vi "Main.vi"() -> ()   [LabVIEW 2020]
doc: "This template is for the Queued Message Handler design pattern.\n\nThe Event Handling Loop generates messages based on user interface actions.\n\nThe Message Handling Loop processes messages generated by the Event Handling Loop, or by other messages. The messages are string values, so new messages can be added easily to the Message Cases case structure in the Message Handling Loop. Each message cluster can also provide an optional value for Message Data, which is a variant that can be converted to whatever message-specific data is required."
uses:
  controls/UI Data.ctl
  controls/Timer Status.ctl
  <vilib>/Skyline/Message/HTTP Wrapper/NI Skyline Message HTTP.lvclass
  C:/Program Files (x86)/National Instruments/LabVIEW 2020/vi.lib/Skyline/Message/NI Skyline Message.lvclass
  <vilib>/Skyline/Configuration/Configuration HTTP_class/Open Configuration HTTP.vi
  <vilib>/Utility/error.llb/Error Cluster From Error Code.vi
  support/Message Queue/Enqueue Message (Single).vi
  <vilib>/ErrorRing/Error Ring.xnode
  support/Message Queue/Message Queue.lvlib
  support/User Event - Stop/User Event - Stop.lvlib
  <vilib>/Skyline/Configuration/Configuration HTTP_class/NI Skyline Configuration HTTP.lvclass
panel:
  in  "Reset Button":bool
  in  "Pause Button":bool
  in  "Start Button":bool
  out "Running":bool
  out "Timer":dbl format="%.2f"
  in  "Exit":bool
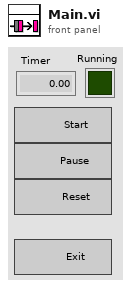
[diagram p1: front panel]
types:
  T1 = typedef "UI Data.ctl" = cluster{"Start":dbl, "Accumulated":dbl, "Running":bool}
  T2 = typedef "Message Queue.lvlib/All Message Queues.ctl" = cluster{"UI":refnum<queue>}
  T3 = typedef "Timer Status.ctl" = cluster{"Elapsed":dbl, "Running":bool}
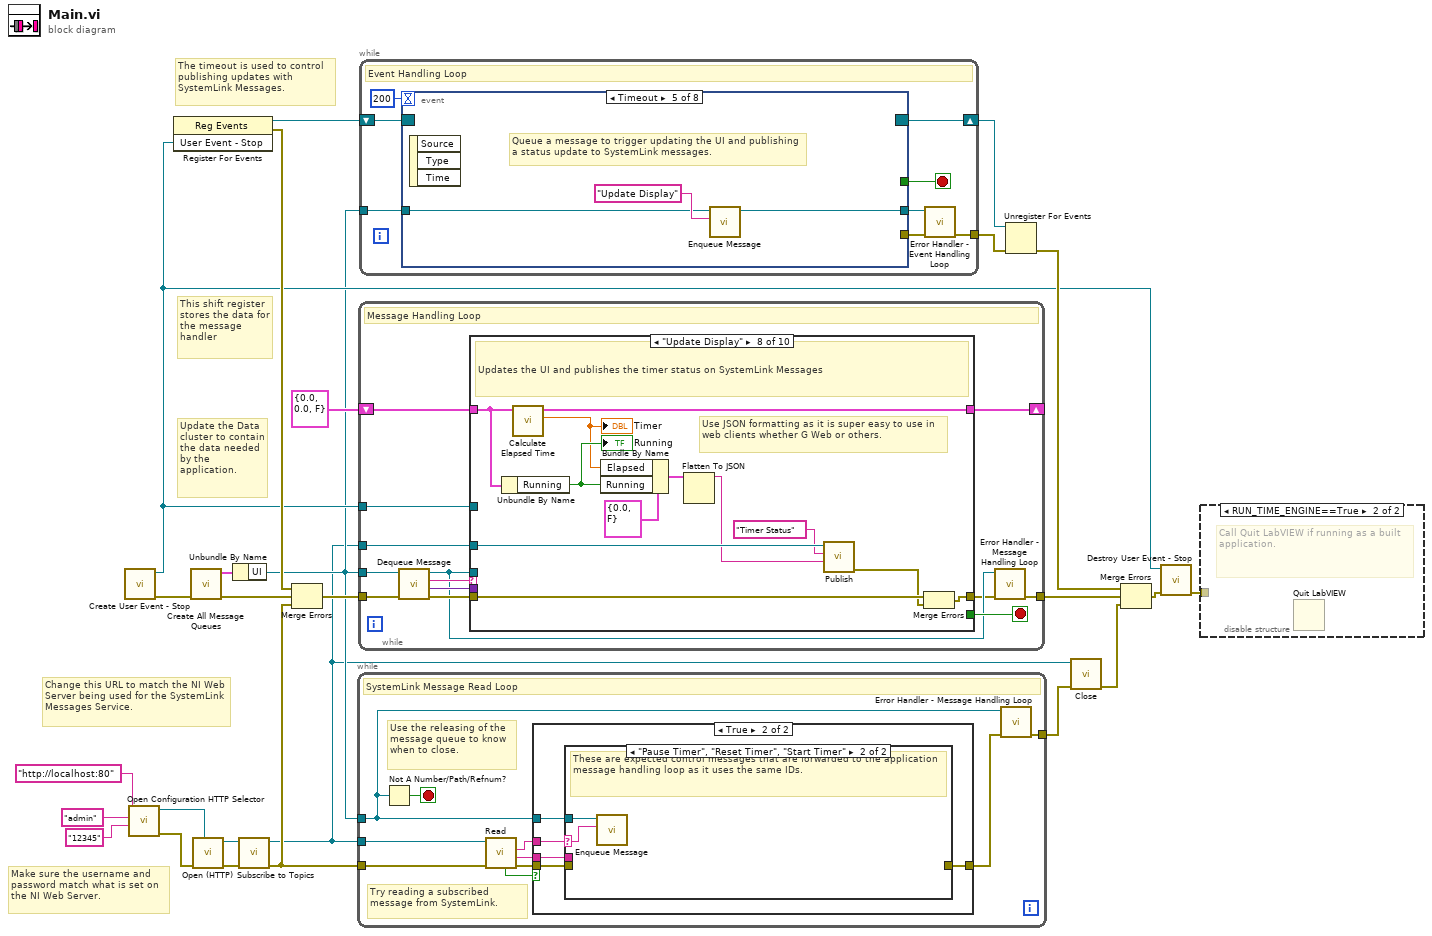
[diagram p0: block diagram]
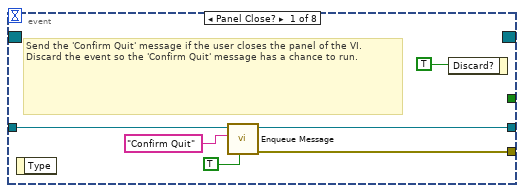
[diagram p3: hidden frame]
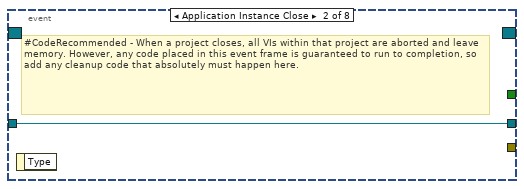
[diagram p4: hidden frame]
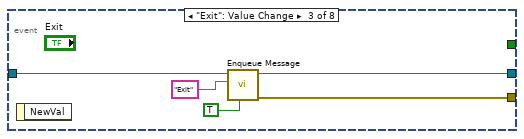
[diagram p5: hidden frame]
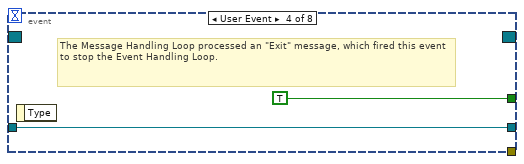
[diagram p6: hidden frame]
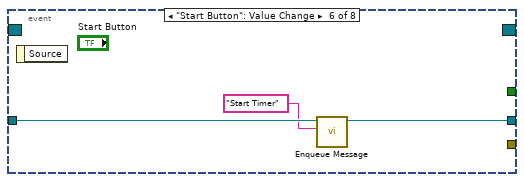
[diagram p7: hidden frame]
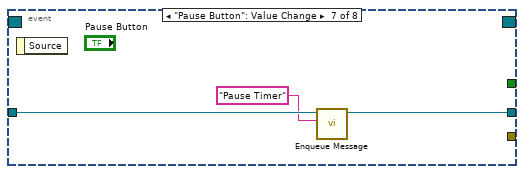
[diagram p8: hidden frame]
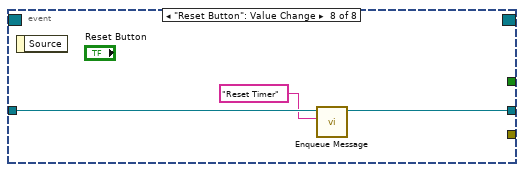
[diagram p9: hidden frame]
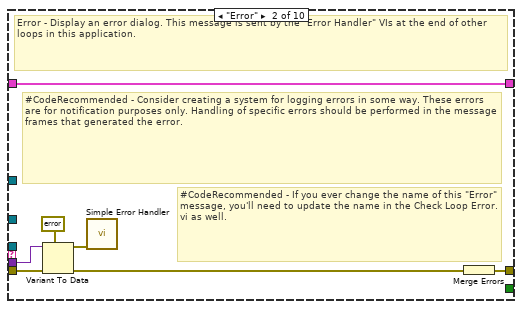
[diagram p11: hidden frame]
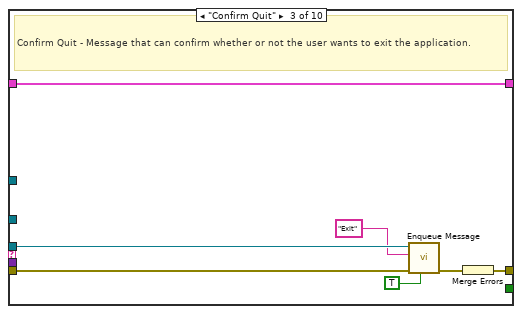
[diagram p12: hidden frame]
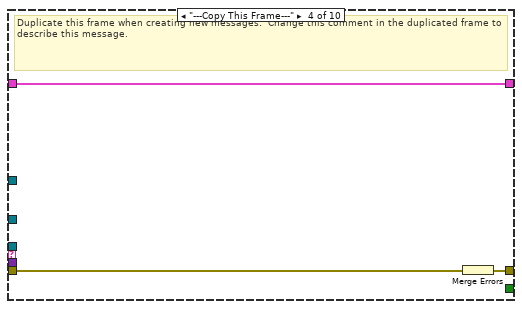
[diagram p13: hidden frame]
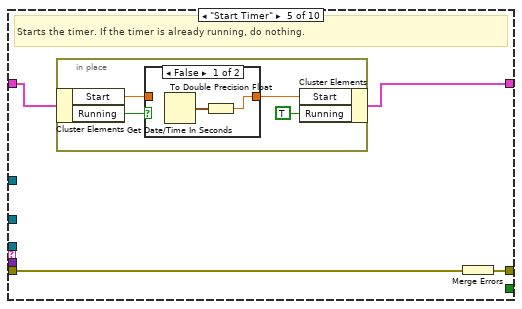
[diagram p14: hidden frame]
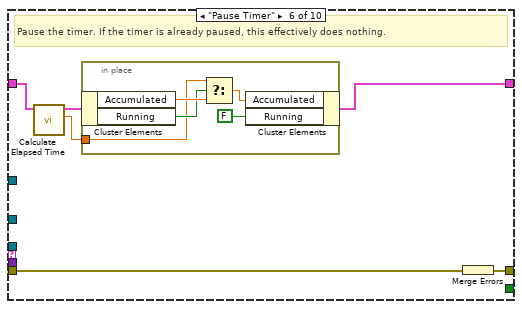
[diagram p16: hidden frame]
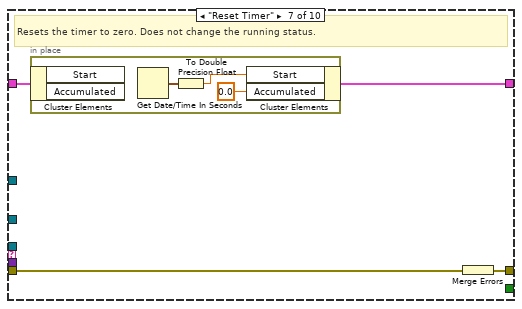
[diagram p17: hidden frame]
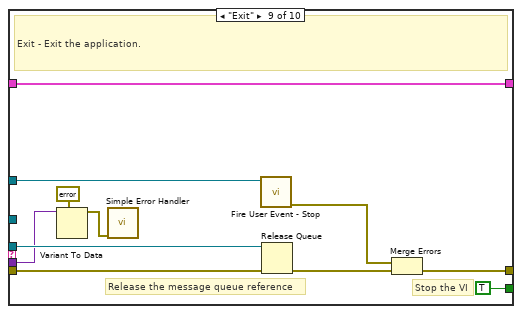
[diagram p18: hidden frame]
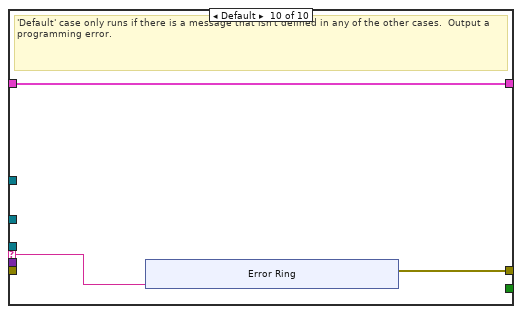
[diagram p19: hidden frame]
diagram:
  # "The timeout is used to control publishing updates with SystemLink Messages."
  # "Update the Data cluster to contain the data needed by the application."
  # "Make sure the username and password match what is set on the NI Web Server."
  # "Change this URL to match the NI Web Server being used for the SystemLink Messages Service."
  # "This shift register stores the data for the message handler"
  n1 = call "Create User Event - Stop.vi"() -> ("error out"=w21:errorcluster, "User Event - Stop"=w13:refnum<user-event>)  [unwired: 10 in]
  n2 = call-poly <vilib>:"Open Configuration HTTP Selector.vi"("password"="12345", "username"="admin", "server url"="http://localhost:80") -> ("error out"=w11:errorcluster, "configuration"=w10:refnum<class "NI Skyline Configuration HTTP.lvclass">)  [unwired: 7 in]
  n3 = register-events(w13) -> (reference out=w14:refnum<event-registration>, error out=w26:errorcluster)  [unwired: 2 in]
  n4 = call "Create All Message Queues.vi"("error in (no error)"=w21) -> ("error out"=w24:errorcluster, "Message Queues out"=w23:T2)  [unwired: 9 in]
  n5 = call <vilib>:"Open (HTTP).vi"("configuration"=w10, "error in (no error)"=w11) -> ("error out"=w6:errorcluster, "message session"=w5:refnum<class "NI Skyline Message HTTP.lvclass">)  [unwired: 8 in]
  n6 = Unbundle By Name(w23) -> ("UI"=w2:refnum<queue>)
  n7 = call "Subscribe to Topics.vi"("error in (no error)"=w6, "message session in"=w5) -> ("error out"=w25:errorcluster, "message session out"=w1:refnum<class "NI Skyline Message HTTP.lvclass">)  [unwired: 8 in]
  n8 = Merge Errors(w26, w24, w25) -> (w12:errorcluster)
  n9 = while {
    tunnel: w2 -> [w28]
    tunnel: w1 -> [w36]
    tunnel: w25 -> [w35]
    tunnel: [w29] -> w4
    stop <- w27 stop-if-true
    # "Try reading a subscribed message from SystemLink."
    # "Use the releasing of the message queue to know when to close."
    # "SystemLink Message Read Loop"
    n10 = Not A Number/Path/Refnum?(number/path/refnum=w28) -> (NaN/Path/Refnum?=w27:bool)
    n11 = call-dynamic "Read.vi"("error in (no error)"=w35, "sync message session in"=w36) -> ("error out"=w31:errorcluster, "message"=w32:string, "topic"=w33:string, "dequeue status"=w34:bool)  [unwired: 5 in, 1 out]
    n12 = case shown="True" w34 {
      tunnel: w33 -> [_ w42]
      tunnel: w32 -> [_ w41]
      tunnel: w28 -> [_ w40]
      tunnel: w31 -> [w37 w39]
      tunnel: [w37 w38] -> w30
      frame False {
        # "No message was received on a topic that's subscribed to, just iterate or possible handle the error that may have been returned from Read.vi"
      }
      frame True {
        n13 = case shown="\"Pause Timer\", \"Reset Timer\", \"Start Timer\"" w42 {
          selector: w42 -> [w43 w52]
          tunnel: w41 -> [_ _]
          tunnel: w40 -> [_ w53]
          tunnel: w39 -> [_ _]
          tunnel: [w44 _] -> w38
          frame Default {
            # "An unrecognized message topic was received. Since we subscribe to specific messages generate an error for the developer to fix."
            n14 = xnode "Error Ring"("parameter 0"=w43) -> ("error out"=w44:errorcluster)
          }
          frame "Pause Timer", "Reset Timer", "Start Timer" {
            # "These are expected control messages that are forwarded to the application message handling loop as it uses the same IDs."
            n15 = call-poly "Enqueue Message.vi"("Message"=w52, "Message Queue"=w53) -> ()  [unwired: 8 in, 2 out]
          }
        }
      }
    }
    n16 = call "Error Handler - Message Handling Loop.vi"("error in (no error)"=w30, "Message Queue"=w28) -> ("dup error in"=w29:errorcluster)  [unwired: 8 in, 1 out]
  }
  n17 = while {
    tunnel: w2 -> [w58]
    shift-right: [w65] -> _
    shift-left: T1 {"Start"=0.0, "Accumulated"=0.0, "Running"=FALSE} ("Data Cluster") -> [w66]
    tunnel: w13 -> [w63]
    tunnel: w12 -> [w62]
    tunnel: [w56] -> w22
    tunnel: w1 -> [w54]
    stop <- w64 stop-if-true
    # "Message Handling Loop"
    n18 = call "Dequeue Message.vi"("error in (no error)"=w62, "Message Queue"=w58) -> ("error out"=w61:errorcluster, "Message Data"=w59:variant, "Message"=w60:string, "dup Message Queue"=w57:refnum<queue>)  [unwired: 6 in]
    n19 = case "Message Cases" shown="\"Update Display\"" w60 {
      selector: w60 -> [_ _ _ _ _ _ _ _ _ w138]
      tunnel: w57 -> [_ _ w78 _ _ _ _ _ w137 _]
      tunnel: w61 -> [w67 w75 w82 w85 w89 w102 w111 w126 w131 _]
      tunnel: [w67 w69 w80 w83 w88 w101 w110 w125 w134 w139] -> w55
      tunnel: w66 -> [w68 w74 w81 w84 w87 w100 w109 w122 w127 w140]
      tunnel: [w68 w74 w81 w84 w86 w97 w108 w123 w127 w140] -> w65
      tunnel: [_ _ _ _ _ _ _ _ TRUE _] -> w64
      tunnel: w59 -> [_ w73 _ _ _ _ _ _ w128 _]
      tunnel: w63 -> [_ _ _ _ _ _ _ _ w133 _]
      tunnel: w54 -> [_ _ _ _ _ _ _ w124 _ _]
      frame "Initialize" {
        # "Initialize - All initialization work should take place in this message, since other loops can potentially enqueue messages that execute immediately after this one."
      }
      frame "Error" {
        # "#CodeRecommended - If you ever change the name of this \"Error\" message, you'll need to update the name in the Check Loop Error.vi as well."
        # "#CodeRecommended - Consider creating a system for logging errors in some way. These errors are for notification purposes only. Handling of specific errors should be performed in the message frames that generated the error."
        # "Error - Display an error dialog. This message is sent by the \"Error Handler\" VIs at the end of other loops in this application."
        n20 = Variant To Data(error in=w75, type=errorcluster {"status"=FALSE, "code"=0, "source"=""} ("error constant"), Variant=w73) -> (data=w71:errorcluster, error out=w70:errorcluster)
        n21 = call <vilib>:"Simple Error Handler.vi"("error in (no error)"=w71) -> ()  [unwired: 4 in, 5 out]
        n22 = Merge Errors(w70) -> (w69:errorcluster)
      }
      frame "Confirm Quit" {
        # "Confirm Quit - Message that can confirm whether or not the user wants to exit the application."
        n23 = call-poly "Enqueue Message.vi"("Priority Message? (F)"=TRUE, "error in (no error)"=w82, "Message"="Exit", "Message Queue"=w78) -> ("error out"=w79:errorcluster)  [unwired: 6 in, 1 out]
        n24 = Merge Errors(w79) -> (w80:errorcluster)
      }
      frame "---Copy This Frame---" {
        # "Duplicate this frame when creating new messages.  Change this comment in the duplicated frame to describe this message."
        n25 = Merge Errors(w85) -> (w83:errorcluster)
      }
      frame "Start Timer" {
        # "Starts the timer. If the timer is already running, do nothing."
        n26 = in-place {
          n27 = in-place-cluster #1(w87) -> ("Start"=w92:dbl, "Running"=w93:bool)
          n28 = case shown="False" w93 {
            tunnel: w92 -> [_ w96]
            tunnel: [w94 w96] -> w90
            frame False {
              n29 = Get Date/Time In Seconds() -> (seconds since 1Jan1904=w95:timestamp)
              n30 = To Double Precision Float(number=w95) -> (double precision float=w94:dbl)
            }
            frame True {
            }
          }
          n31 = in-place-cluster #1("Start"=w90, "Running"=TRUE) -> (w86:T1)
        }
        n32 = Merge Errors(w89) -> (w88:errorcluster)
      }
      frame "Pause Timer" {
        # "Pause the timer. If the timer is already paused, this effectively does nothing."
        n33 = call "Calculate Elapsed Time.vi"("UI Data In"=w100) -> ("Elapsed"=w98:dbl, "UI Data"=w99:T1)  [unwired: 9 in]
        n34 = in-place {
          in-place-border: w98 -> [w105]
          n35 = in-place-cluster #2(w99) -> ("Accumulated"=w107:dbl, "Running"=w106:bool)
          n36 = Select(t=w105, s=w106, f=w107) -> (s? t:f=w104:dbl)
          n37 = in-place-cluster #2("Accumulated"=w104, "Running"=FALSE) -> (w97:T1)
        }
        n38 = Merge Errors(w102) -> (w101:errorcluster)
      }
      frame "Reset Timer" {
        # "Resets the timer to zero. Does not change the running status."
        n39 = in-place {
          n40 = in-place-cluster #3(w109) -> ()  [unwired: 2 out]
          n41 = Get Date/Time In Seconds() -> (seconds since 1Jan1904=w114:timestamp)
          n42 = To Double Precision Float(number=w114) -> (double precision float=w113:dbl)
          n43 = in-place-cluster #3("Start"=w113, "Accumulated"=0.0) -> (w108:T1)
        }
        n44 = Merge Errors(w111) -> (w110:errorcluster)
      }
      frame "Update Display" {
        # "Use JSON formatting as it is super easy to use in web clients whether G Web or others."
        # "Updates the UI and publishes the timer status on SystemLink Messages"
        n45 = Unbundle By Name(w122) -> ("Running"=w120:bool)
        "Running" <- w120
        n46 = call "Calculate Elapsed Time.vi"("UI Data In"=w122) -> ("Elapsed"=w119:dbl, "UI Data"=w123:T1)  [unwired: 9 in]
        "Timer" <- w119
        n47 = Bundle By Name(cluster=T3 {"Elapsed"=0.0, "Running"=FALSE} ("Timer Status"), "Elapsed"=w119, "Running"=w120) -> (w118:T3)
        n48 = Flatten To JSON(anything=w118) -> (JSON string=w117:string)  [unwired: 2 in, 1 out]
        n49 = call-dynamic "Publish.vi"("message"=w117, "topic"="Timer Status", "message session in"=w124) -> ("error out"=w115:errorcluster)  [unwired: 7 in, 1 out]
        n50 = Merge Errors(w126, w115) -> (w125:errorcluster)
      }
      frame "Exit" {
        # "Stop the VI"
        # "Release the message queue reference"
        # "Exit - Exit the application."
        n51 = Variant To Data(type=errorcluster {"status"=FALSE, "code"=0, "source"=""} ("error constant"), Variant=w128) -> (data=w129:errorcluster)  [unwired: 1 in, 1 out]
        n52 = call <vilib>:"Simple Error Handler.vi"("error in (no error)"=w129) -> ()  [unwired: 4 in, 5 out]
        n53 = call "Fire User Event - Stop.vi"("User Event - Stop"=w133) -> ("error out"=w132:errorcluster)  [unwired: 10 in]
        n54 = Release Queue(queue=w137, error in (no error)=w131) -> (error out=w135:errorcluster)  [unwired: 1 in, 2 out]
        n55 = Merge Errors(w132, w135) -> (w134:errorcluster)
      }
      frame Default {
        # "'Default' case only runs if there is a message that isn't defined in any of the other cases.  Output a programming error."
        n56 = xnode "Error Ring"("parameter 0"=w138) -> ("error out"=w139:errorcluster)
      }
    }
    n57 = call "Error Handler - Message Handling Loop.vi"("error in (no error)"=w55, "Message Queue"=w57) -> ("dup error in"=w56:errorcluster)  [unwired: 8 in, 1 out]
  }
  n58 = while {
    tunnel: w2 -> [w155]
    shift-right: [w153] -> w18
    shift-left: w14 -> [w154]
    tunnel: [w149] -> w15
    stop <- w151 stop-if-true
    # "Event Handling Loop"
    n59 = event shown="[4] Timeout" {
      selector: w154 -> [_ _ _ _ _ _ _ _]
      dyn-events: [_ _ _ _ _ _ _ _] -> w153
      timeout: 200 -> [_ _ _ _ _ _ _ _]
      tunnel: [_ _ _ TRUE ("Discard?") _ _ _ _] -> w151
      tunnel: w155 -> [w160 w162 w167 w169 w170 w175 w178 w181]
      tunnel: [w159 _ w166 _ _ _ _ _] -> w152
      tunnel: [w158 w162 w165 w169 w172 w174 w177 w180] -> w150
      event Panel Close? {
        # "Send the 'Confirm Quit' message if the user closes the panel of the VI. Discard the event so the 'Confirm Quit' message has a chance to run."
        n60 = event-data() -> ()  [unwired: 1 in, 1 out]
        n61 = call-poly "Enqueue Message.vi"("Priority Message? (F)"=TRUE, "Message"="Confirm Quit", "Message Queue"=w160) -> ("error out"=w159:errorcluster, "dup Message Queue"=w158:refnum<queue>)  [unwired: 7 in]
        n62 = event-data("Discard?"=TRUE) -> ()  [unwired: 1 in, 1 out]
      }
      event Application Instance Close {
        # "#CodeRecommended - When a project closes, all VIs within that project are aborted and leave memory. However, any code placed in this event frame is guaranteed to run to completion, so add any cleanup code that absolutely must happen here."
        n63 = event-data() -> ()  [unwired: 1 in, 1 out]
      }
      event "Exit": Value Change {
        n64 = event-data() -> ()  [unwired: 1 in, 1 out]
        n65 = call-poly "Enqueue Message.vi"("Priority Message? (F)"=TRUE, "Message"="Exit", "Message Queue"=w167) -> ("error out"=w166:errorcluster, "dup Message Queue"=w165:refnum<queue>)  [unwired: 7 in]
      }
      event User Event {
        # "The Message Handling Loop processed an \"Exit\" message, which fired this event to stop the Event Handling Loop."
        n66 = event-data() -> ()  [unwired: 1 in, 1 out]
      }
      event Timeout {
        # "Queue a message to trigger updating the UI and publishing a status update to SystemLink messages."
        n67 = event-data() -> ()  [unwired: 1 in, 3 out]
        n68 = call-poly "Enqueue Message.vi"("Message"="Update Display", "Message Queue"=w170) -> ("dup Message Queue"=w172:refnum<queue>)  [unwired: 8 in, 1 out]
      }
      event "Start Button": Value Change {
        n69 = event-data() -> ()  [unwired: 1 in, 1 out]
        n70 = call-poly "Enqueue Message.vi"("Message"="Start Timer", "Message Queue"=w175) -> ("dup Message Queue"=w174:refnum<queue>)  [unwired: 8 in, 1 out]
      }
      event "Pause Button": Value Change {
        n71 = event-data() -> ()  [unwired: 1 in, 1 out]
        n72 = call-poly "Enqueue Message.vi"("Message"="Pause Timer", "Message Queue"=w178) -> ("dup Message Queue"=w177:refnum<queue>)  [unwired: 8 in, 1 out]
      }
      event "Reset Button": Value Change {
        n73 = event-data() -> ()  [unwired: 1 in, 1 out]
        n74 = call-poly "Enqueue Message.vi"("Message"="Reset Timer", "Message Queue"=w181) -> ("dup Message Queue"=w180:refnum<queue>)  [unwired: 8 in, 1 out]
      }
    }
    n75 = call "Error Handler - Event Handling Loop.vi"("error in (no error)"=w152, "Message Queue"=w150) -> ("dup error in"=w149:errorcluster)  [unwired: 8 in, 1 out]
  }
  n76 = Unregister For Events(event registration refnum=w18, error in=w15) -> (error out=w19:errorcluster)
  n77 = call-dynamic "Close.vi"("error in (no error)"=w4, "message session"=w1) -> ("error out"=w3:errorcluster)  [unwired: 9 in]
  n78 = Merge Errors(w19, w22, w3) -> (w20:errorcluster)
  n79 = call "Destroy User Event - Stop.vi"("error in (no error)"=w20, "User Event - Stop"=w13) -> ("error out"=w16:errorcluster)  [unwired: 9 in]
  n80 = disable-structure shown="RUN_TIME_ENGINE==True" {
    disable-tunnel: w16 -> [_ _]
    frame condition #0 (active) {
    }
    frame condition #1 {
      # "Call Quit LabVIEW if running as a built application."
      n81 = Quit LabVIEW() -> ()  [unwired: 1 in]
    }
  }
